vi "create queue connection.vi"(8 "error in":errorcluster, 10 "queues":T1) -> (0 "error out":errorcluster, 3 "TCP connection out":refnum<class "Queue connection.lvclass">)   [LabVIEW 2015, in "Queue connection.lvclass"]
uses:
  Queue connection.lvclass
  queue pair.ctl
  message/communicator message.lvclass
  Queue connection.lvclass/Queue connection.ctl
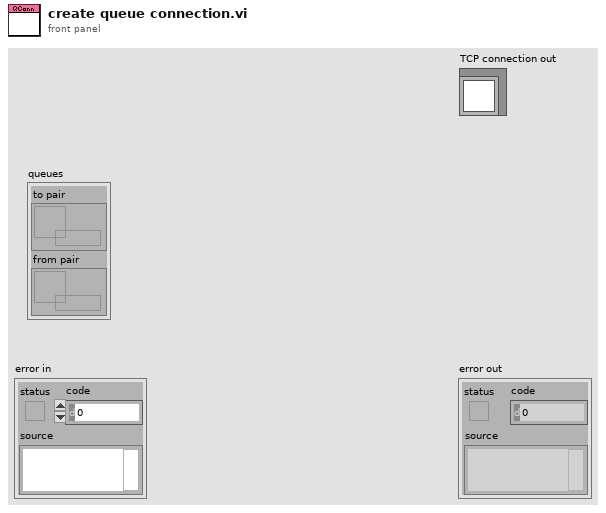
[diagram p1: front panel]
types:
  T1 = typedef "Queue connection.lvclass/queue pair.ctl" = cluster{"to pair":refnum<queue>, "from pair":refnum<queue>}
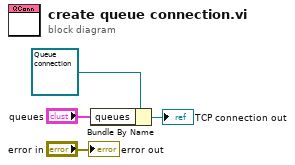
[diagram p0: block diagram]
diagram:
  n1 = Bundle By Name(cluster=refnum<class "Queue connection.lvclass"> refnum ("TCP connection in"), "queues"="queues") -> (→"TCP connection out":refnum<class "Queue connection.lvclass">)
  "error out" <- "error in"
